vi "MHM error coding.vi"(8 "error in (no error)":errorcluster, 11 "function return in":u32) -> (0 "error out":errorcluster)   [LabVIEW 2017, in "MHM_1SL_interface.lvlib"]
uses:
  MHM_1SL_interface.lvlib
  enums/MHM_ErrorEnum.ctl
panel:
  in  "MHM_ErrorEnum":T1
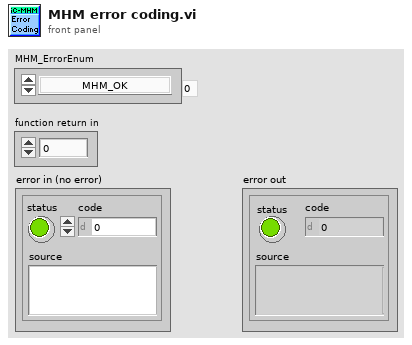
[diagram p1: front panel]
types:
  T1 = typedef "MHM_ErrorEnum.ctl" = enum16{"MHM_OK", "MHM_INVALID_HANDLE", "MHM_INTERFACEDRIVER_NOT_FOUND", "MHM_INTERFACE_NOT_FOUND", "MHM_INVALID_INTERFACE", "MHM_INVALID_PARAMETER", "MHM_INVALID_ADDRESS", "MHM_INVALID_VALUE", "MHM_USB_ERROR", "MHM_FILE_NOT_FOUND", "MHM_INVALID_FILE", "MHM_VERIFY_FAILED", "MHM_MASTERCOMM_FAILED", "MHM_BISSCOMM_FAILED", "MHM_SPICOMM_FAILED", "MHM_USB_HIGHSPEED_WARNING", "MHM_INVALID_BISSMASTER", "MHM_NO_INTERFACE_SELECTED", "MHM_READPARAM_SSI", "MHM_SPI_ERROR", "MHM_SPI_DISMISS", "MHM_SPI_FAIL", "MHM_SPI_BUSY_TIMEOUT", "MHM_FILE_ACCESS_DENIED", "MHM_INVALID_CONFIGURATION", "MHM_INVALID_EDS", "MHM_INVALID_EDS_CHCKSUM", "MHM_EDS_CORRECTED", "MHM_CORRECTED_INVALID_VALUE", "MHM_BISS_REGERROR", "MHM_EDS_UNDEFINED", "MHM_FILESIZE_WARNING", "MHM_SLOW_ROTATION", "MHM_FAST_ROTATION", "MHM_GAIN_LIMIT", "MHM_ACQUISITION_FAILED", "MHM_USB_DATA_LOSS", "MHM_INTERNAL_CALIB_ERROR", "MHM_OFFSET_LIMIT", "MHM_CALIBRATION_FAILED", "MHM_I2C_COMM_FAILED", "MHM_GAINCOSCORR_LIMIT", "MHM_HARMCAL_LIMIT", "MHM_BAD_CAL_DATA"}
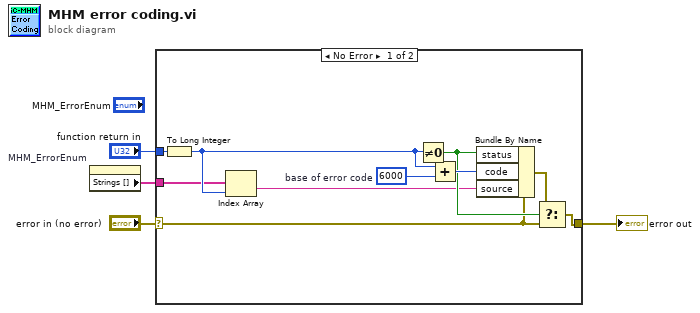
[diagram p0: block diagram]
diagram:
  n1 = property on="MHM_ErrorEnum" class="Enum (strict)"() -> ("Strings []"=w1:string[])  [unwired: 2 in, 2 out]
  n2 = case shown="No Error" "error in (no error)" {
    selector: "error in (no error)" -> [w9 w15]
    tunnel: [w8 w15] -> w3
    tunnel: "function return in" -> [w13 _]
    tunnel: w1 -> [w6 _]
    frame No Error {
      w14 = 6000  # base of error code
      n3 = To Long Integer(number=w13) -> (32bit integer=w7:i32)
      n4 = Index Array(array=w6, index=w7) -> (element=w5:string)
      n5 = Not Equal To 0?(x=w7) -> (x != 0?=w11:bool)
      n6 = Add(x=w7, y=w14) -> (x+y=w12:i32)
      n7 = Bundle By Name(cluster=w9, "status"=w11, "code"=w12, "source"=w5) -> (w10:errorcluster)
      n8 = Select(t=w10, s=w11, f=w9) -> (s? t:f=w8:errorcluster)
    }
    frame Error {
    }
  }
  "error out" <- w3
